vi "Get Finite Analog Sample.vi"(0 "Arduino Resource":T1={"VISA resource"="", "Board Type"=enum."Uno", "Connection Type"=enum."USB / Serial", "Bytes Per Packet (15)"=15}, 1 "Analog Input Pin":u8, 2 "Acquition Speed (HZ)":u16, 3 "Number of Samples":u16, 5 "error in":errorcluster) -> (14 "Arduino Resource":T1={"VISA resource"="", "Board Type"=enum."Uno", "Connection Type"=enum."USB / Serial", "Bytes Per Packet (15)"=15}, 15 "Samples Aquired":i32, 16 "Data":waveform(dbl)(graph), 19 "error out":errorcluster)   [LabVIEW 2015, in "LabVIEW Interface for Arduino.lvlib"]
doc: "Acquire a finite number of samples from the specified analog input pin at the user specified rate (up to 5Khz)"
uses:
  <vilib>/LabVIEW Interface for Arduino/LabVIEW Interface for Arduino.lvlib
  <vilib>/LabVIEW Interface for Arduino/Type Defs/Arduino Resource.ctl
  <vilib>/LabVIEW Interface for Arduino/Type Defs/Board Type.ctl
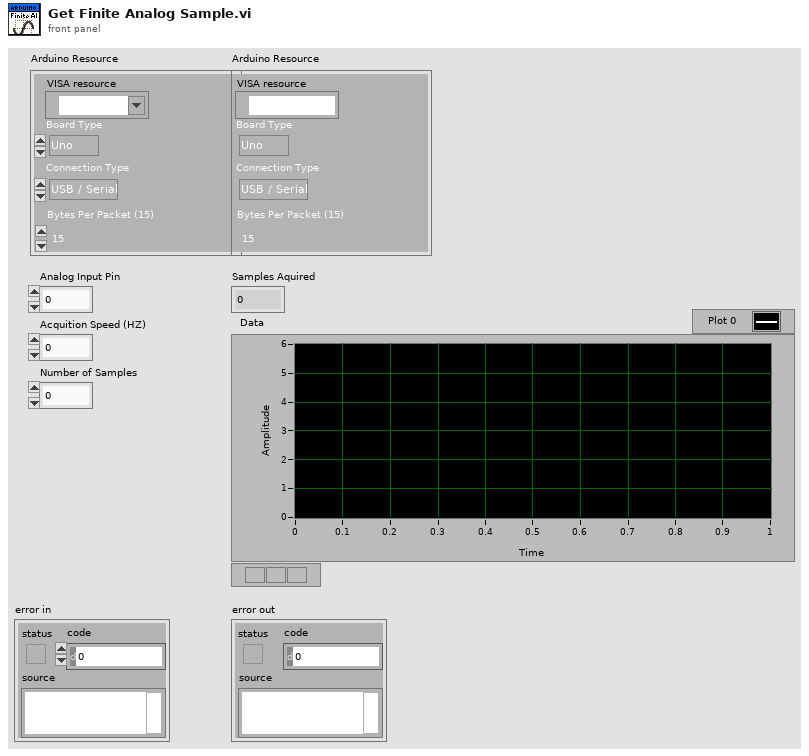
[diagram p1: front panel]
types:
  T1 = typedef "LabVIEW Interface for Arduino.lvlib/Arduino Resource.ctl" = cluster{"VISA resource":refnum<visa-resource-name>, "Board Type":T2, "Connection Type":enum8{"USB / Serial"}, "Bytes Per Packet (15)":u8}
  T2 = typedef "LabVIEW Interface for Arduino.lvlib/Board Type.ctl" = enum16{"Uno", "Dimuelanove w/Atmega 328", "Mega 2560"}
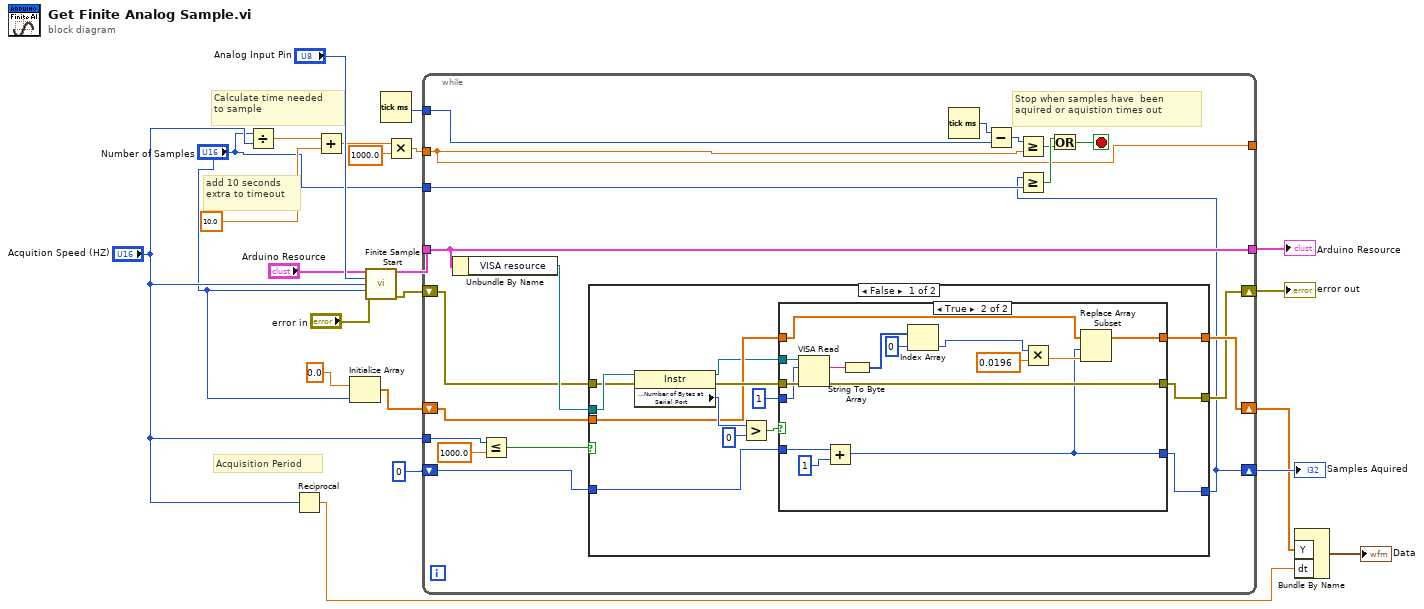
[diagram p0: block diagram]
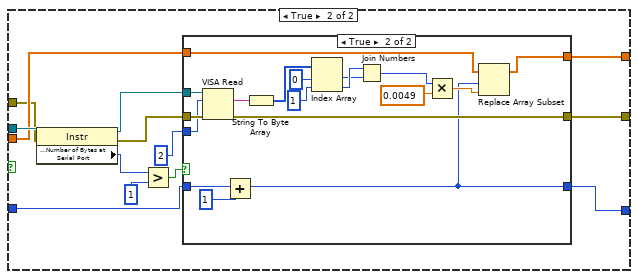
[diagram p3: hidden frame]
diagram:
  # "Calculate time needed\nto sample"
  # "Acquisition Period"
  # "add 10 seconds\nextra to timeout"
  n1 = Divide(x="Number of Samples", y="Acquition Speed (HZ)") -> (x/y=w15:dbl)
  n2 = Reciprocal(x="Acquition Speed (HZ)") -> (1/x=w7:dbl)
  n3 = Add(x=w15, y=10.0) -> (x+y=w16:dbl)
  n4 = Initialize Array(0.0 ("element"), "Number of Samples") -> (w9:dbl[])
  n5 = call <vilib>:"Finite Sample Start.vi"("Arduino Resource"="Arduino Resource", "Analog Input Pin"="Analog Input Pin", "Acquition Speed (HZ)"="Acquition Speed (HZ)", "Number of Samples"="Number of Samples", "error in"="error in") -> ("Arduino Resource"=w21:T1, "error out"=w20:errorcluster)  [unwired: 9 in]
  n6 = Tick Count (ms)() -> (millisecond timer value=w19:u32)
  n7 = Multiply(x=w16, y=1000.0) -> (x*y=w14:dbl)
  n8 = while {
    shift-right: [w23] -> w12
    shift-left: 0 -> [w31]
    tunnel: w21 -> [w41]
    tunnel: [w41] -> w5
    shift-right: [w27] -> w3
    shift-left: w20 -> [w29]
    tunnel: "Number of Samples" -> [w40]
    tunnel: w19 -> [w38]
    tunnel: w14 -> [w33]
    tunnel: [w33] -> _
    shift-right: [w28] -> w8
    shift-left: w9 -> [w30]
    tunnel: "Acquition Speed (HZ)" -> [w24]
    stop <- w34 stop-if-true
    # "Stop when samples have  been \naquired or aquistion times out"
    n9 = Unbundle By Name(w41) -> ("VISA resource"=w32:refnum<visa-resource-name>)
    n10 = Less Or Equal?(x=w24, y=1000.0) -> (x <= y?=w26:bool)
    n11 = case shown="False" w26 {
      tunnel: [w48 w85] -> w23
      tunnel: [w49 w83] -> w27
      tunnel: w32 -> [w46 w78]
      tunnel: w31 -> [w47 w77]
      tunnel: w30 -> [w43 w76]
      tunnel: w29 -> [w45 w73]
      tunnel: [w44 w75] -> w28
      frame False {
        n12 = property class="Instr"(reference=w46, error in=w45) -> (reference out=w42:refnum<visa-resource-name>, error out=w50:errorcluster, "Serial Settings:Number of Bytes at Serial Port"=w51:u32)
        n13 = Greater?(x=w51, y=u32 0) -> (0:w54:bool)
        n14 = case shown="True" w54 {
          tunnel: [w56 w61] -> w48
          tunnel: w50 -> [w57 w72]
          tunnel: [w57 w71] -> w49
          tunnel: 1 -> [_ w70]
          tunnel: w47 -> [w56 w63]
          tunnel: [w55 w60] -> w44
          tunnel: w43 -> [w55 w59]
          tunnel: w42 -> [_ w58]
          frame False {
          }
          frame True {
            n15 = VISA Read(VISA resource name=w58, byte count=w70, error in (no error)=w72) -> (read buffer=w69:string, error out=w71:errorcluster)  [unwired: 2 out]
            n16 = Add(x=w63, y=1) -> (x+y=w61:i32)
            n17 = String To Byte Array(string=w69) -> (unsigned byte array=w68:u8[])
            n18 = Index Array(array=w68, index=0) -> (element=w64:u8)
            n19 = Multiply(x=w64, y=0.0196) -> (x*y=w62:dbl)
            n20 = Replace Array Subset(array=w59, new element=w62, index=w61) -> (w60:dbl[])
          }
        }
      }
      frame True {
        n21 = property class="Instr"(reference=w78, error in=w73) -> (reference out=w74:refnum<visa-resource-name>, error out=w84:errorcluster, "Serial Settings:Number of Bytes at Serial Port"=w82:u32)
        n22 = Greater?(x=w82, y=u32 1) -> (0:w79:bool)
        n23 = case shown="True" w79 {
          tunnel: [w87 w92] -> w85
          tunnel: w84 -> [w88 w106]
          tunnel: [w88 w105] -> w83
          tunnel: 2 -> [_ w104]
          tunnel: [w86 w90] -> w75
          tunnel: w77 -> [w87 w94]
          tunnel: w76 -> [w86 w91]
          tunnel: w74 -> [_ w89]
          frame False {
          }
          frame True {
            n24 = VISA Read(VISA resource name=w89, byte count=w104, error in (no error)=w106) -> (read buffer=w103:string, error out=w105:errorcluster)  [unwired: 2 out]
            n25 = Add(x=w94, y=1) -> (x+y=w92:i32)
            n26 = String To Byte Array(string=w103) -> (unsigned byte array=w102:u8[])
            n27 = Index Array(array=w102, index #1=0 ("index"), index #2=1 ("index")) -> (element #1=w96:u8, element #2=w97:u8)
            n28 = Join Numbers(hi=w97, lo=w96) -> ((hi.lo)=w95:u16)
            n29 = Multiply(x=w95, y=0.0049) -> (x*y=w93:dbl)
            n30 = Replace Array Subset(array=w91, new element=w93, index=w92) -> (w90:dbl[])
          }
        }
      }
    }
    n31 = Tick Count (ms)() -> (millisecond timer value=w37:u32)
    n32 = Subtract(x=w37, y=w38) -> (x-y=w36:u32)
    n33 = Greater Or Equal?(x=w36, y=w33) -> (x >= y?=w35:bool)
    n34 = Greater Or Equal?(x=w23, y=w40) -> (x >= y?=w39:bool)
    n35 = Or(x=w39, y=w35) -> (x .or. y?=w34:bool)
  }
  "Samples Aquired" <- w12
  "Arduino Resource" <- w5
  "error out" <- w3
  n36 = Bundle By Name("Y"=w8, "dt"=w7) -> (→"Data":waveform(dbl))  [unwired: 1 in]
